vi "mesageUserEvent.vi"() -> ()   [LabVIEW 2015]
panel:
  in  "stop":bool
  in  "String":string
  in  "Boolean":bool
  out "Moje zdarzenie":string
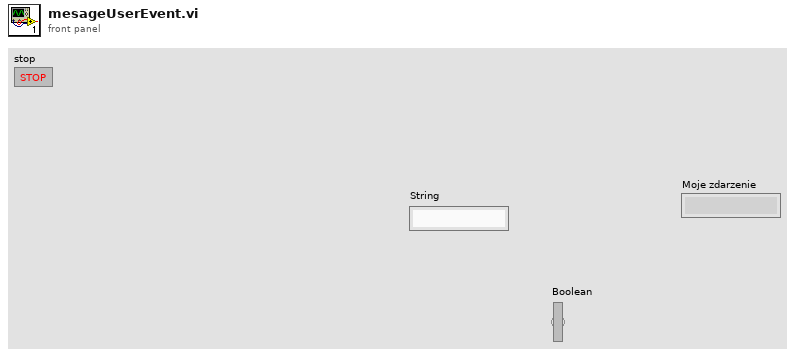
[diagram p1: front panel]
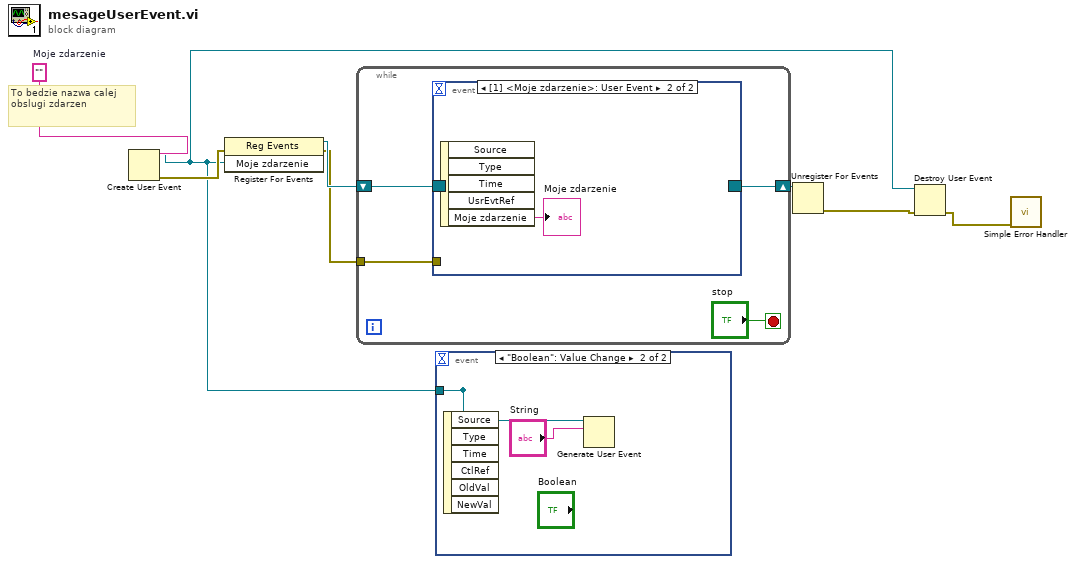
[diagram p0: block diagram]
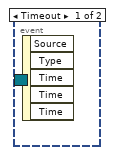
[diagram p2: hidden frame]
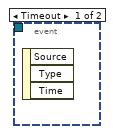
[diagram p3: hidden frame]
diagram:
  w8 = ""  # Moje zdarzenie
  # "To bedzie nazwa calej obslugi zdarzen"
  n1 = Create User Event(user event datatype=w8) -> (user event=w1:refnum<user-event>, error out=w4:errorcluster)  [unwired: 1 in]
  n2 = register-events(error in=w4, w1) -> (reference out=w7:refnum<event-registration>, error out=w3:errorcluster)  [unwired: 1 in]
  n3 = while {
    tunnel: w3 -> [w10]
    shift-right: [w11] -> w6
    shift-left: w7 -> [w12]
    stop <- "stop" stop-if-true
    n4 = event shown="[1] <Moje zdarzenie>: User Event" {
      selector: w12 -> [_ _]
      dyn-events: [_ _] -> w11
      timeout: _ -> [_ _]
      tunnel: w10 -> [_ _]
      event Timeout {
        n5 = event-data() -> ()  [unwired: 1 in, 5 out]
      }
      event User Event {
        n6 = event-data() -> ("Moje zdarzenie"=→"Moje zdarzenie":string)  [unwired: 1 in, 4 out]
      }
    }
  }
  n7 = event shown="[1] \"Boolean\": Value Change" {
    selector: _ -> [_ _]
    dyn-events: _ -> [_ _]
    timeout: _ -> [_ _]
    tunnel: [_ w15] -> _
    tunnel: w1 -> [_ w15]
    event Timeout {
      n8 = event-data() -> ()  [unwired: 1 in, 3 out]
    }
    event "Boolean": Value Change {
      n9 = event-data() -> ()  [unwired: 1 in, 6 out]
      n10 = Generate User Event(user event=w15, event data cluster="String") -> ()  [unwired: 2 in, 2 out]
    }
  }
  n11 = Unregister For Events(event registration refnum=w6) -> (error out=w5:errorcluster)  [unwired: 1 in]
  n12 = Destroy User Event(user event=w1, error in=w5) -> (error out=w2:errorcluster)
  n13 = call <vilib>:"Simple Error Handler.vi"("error in (no error)"=w2) -> ()  [unwired: 4 in, 5 out]
